vi "valves.vi"() -> ()   [LabVIEW 2012]
panel:
  in  "odor 2":bool
  in  "odor 1":bool
  in  "control stream":bool
  out "valves":bool[](array[boolean])
  in  "stop":bool
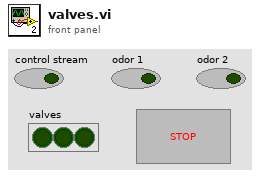
[diagram p1: front panel]
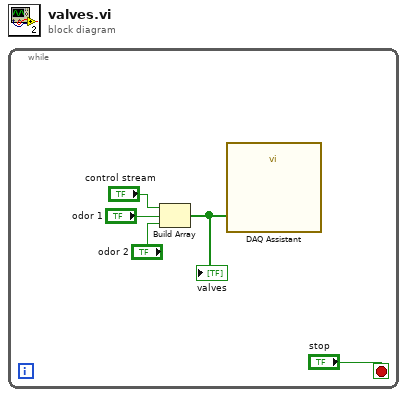
[diagram p0: block diagram]
diagram:
  n1 = while {
    stop <- "stop" stop-if-true
    n2 = Build Array("control stream", "odor 1", "odor 2") -> (w1:bool[])
    "valves" <- w1
    n3 = call "DAQ Assistant"("data"=w1) -> ()  [unwired: 17 in, 2 out]
  }
